vi "generate default line.vi"(8 "error in":errorcluster, 11 "operations table":T2) -> (0 "error out":errorcluster, 2 "line item in":T1)   [LabVIEW 2013, in "Scan Engine editor node.lvclass"]
uses:
  Scan Engine editor node.lvclass
  table reference.ctl
  table line.ctl
  <vilib>/NI/Tag Bus Module Framework/channel/TBM channel.lvclass
  <vilib>/NI/Tag Bus/tag/Data Type.ctl
  permissions.ctl
  <vilib>/NI/Tag Bus/tag/tag descriptor.lvclass/tag descriptor.ctl
  <vilib>/NI/Tag Bus/tag/tag descriptor.lvclass
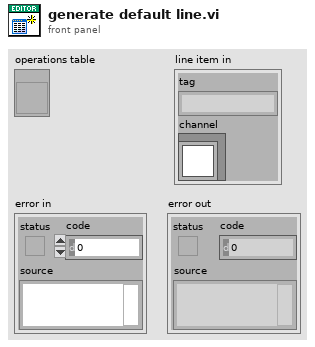
[diagram p1: front panel]
types:
  T1 = typedef "Scan Engine editor node.lvclass/table line.ctl" = cluster{"tag":string, "channel":refnum<class "TBM channel.lvclass">}
  T2 = typedef "Scan Engine editor node.lvclass/table reference.ctl" = refnum<vi>
  T3 = typedef "Scan Engine editor node.lvclass/permissions.ctl" = enum32{"Read from HW", "Write to HW"}
  T4 = typedef "tag bus.lvlib/tag descriptor.lvclass/Data Type.ctl" = enum16{"Double", "Single", "I64", "I32", "I16", "I8", "U64", "U32", "U16", "U8", "Boolean", "String", "Array of Double", "Array of Single", "Array of I64", "Array of I32", "Array of I16", "Array of I8", "Array of U64", "Array of U32", "Array of U16", "Array of U8", "Array of Boolean", "Array of String"}
  T5 = typedef "TBM channel.lvclass/channel classification.ctl" = enum16{"input data", "output data", "processing parameter", "processing result"}
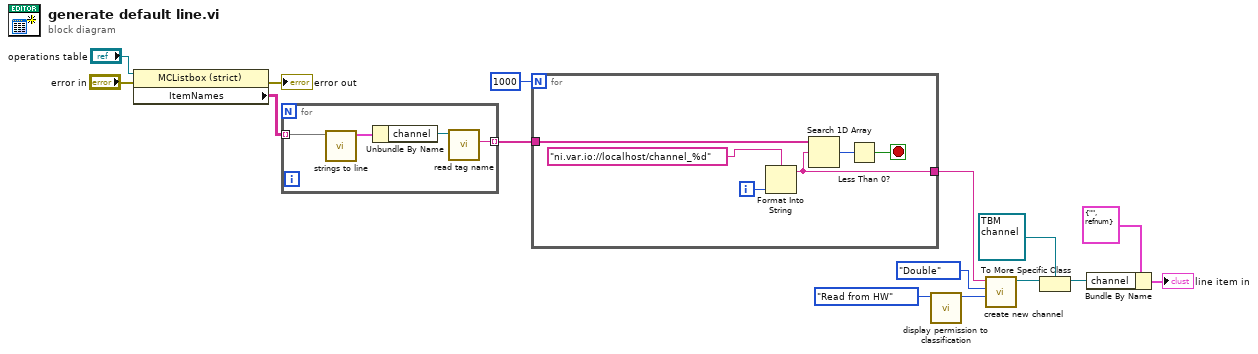
[diagram p0: block diagram]
diagram:
  n1 = property class="MCListbox (strict)"(reference="operations table", error in="error in") -> (error out=→"error out":errorcluster, "ItemNames"=w12:string[][])  [unwired: 1 out]
  n2 = for {
    tunnel: w12 -> [w19] mode=indexing
    tunnel: [w16] -> w10 mode=indexing
    n3 = call "strings to line.vi"("strings"=w19) -> ("line"=w18:T1)  [unwired: 10 in]
    n4 = Unbundle By Name(w18) -> ("channel"=w17:refnum<class "TBM channel.lvclass">)
    n5 = call <vilib>:"read tag name.vi"("system tag in"=w17) -> ("name"=w16:string)  [unwired: 8 in, 2 out]
  }
  n6 = for {
    N: 1000 -> [_]
    tunnel: w10 -> [w23]
    tunnel: [w20] -> w9
    i -> [w25]
    stop <- w21 stop-if-true
    n7 = Format Into String(format string="ni.var.io://localhost/channel_%d", w25) -> (resulting string=w20:string)  [unwired: 2 in, 1 out]
    n8 = Search 1D Array(1D array=w23, element=w20) -> (index of element=w22:i32)  [unwired: 1 in]
    n9 = Less Than 0?(x=w22) -> (x < 0?=w21:bool)
  }
  n10 = call "display permission to classification.vi"("display permissions"=permissions."Read from HW") -> ("channel classification"=w6:T5)  [unwired: 10 in]
  n11 = call <vilib>:"create new channel.vi"("channel classification"=w6, "data type"=Data_Type."Double", "channel name"=w9) -> ("channel"=w3:refnum<class "TBM channel.lvclass">)  [unwired: 8 in]
  n12 = To More Specific Class(target class=refnum<class "TBM channel.lvclass"> refnum ("channel"), reference=w3) -> (specific class reference=w2:refnum<class "TBM channel.lvclass">)  [unwired: 1 in, 1 out]
  n13 = Bundle By Name(cluster=T1 {"tag"="", "channel"=refnum} ("line item in 2"), "channel"=w2) -> (→"line item in":T1)
